vi "Init.vi"(8 "error in (no error)":errorcluster, 11 "Initial Data":string[][](table)=[["Test", "Dummy"], ["Operator", "John"], ["DUT", "Golden"], ["Serial Number", "0xAB"], ["Timestamp", "5/1/2023"]]) -> (0 "error out":errorcluster, 3 "DVR out":refnum<class "Data Server.lvclass">)   [LabVIEW 2021, in "Veristandgrpc_server.lvlib" / "Data Server.lvclass"]
uses:
  Data Server.lvclass
  Data Server.lvclass/Data Server.ctl
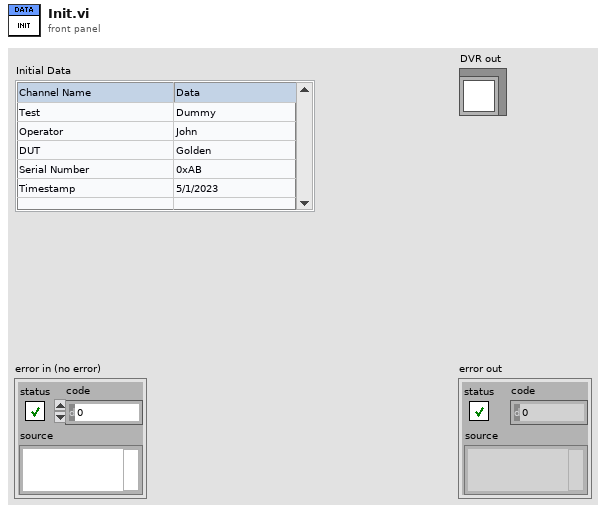
[diagram p1: front panel]
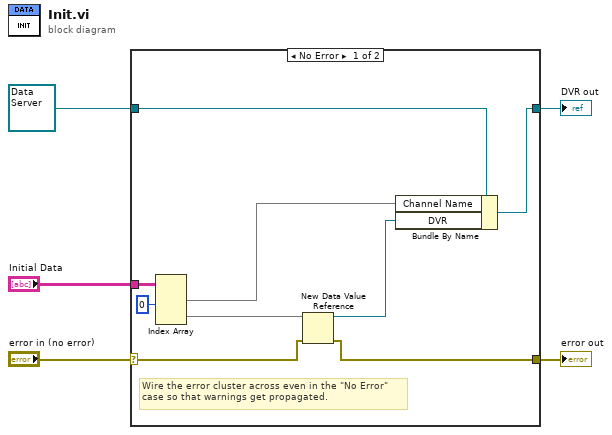
[diagram p0: block diagram]
diagram:
  n1 = case shown="No Error" "error in (no error)" {
    selector: "error in (no error)" -> [w9 w16]
    tunnel: [w7 w16] -> w4
    tunnel: [w13 w15] -> w2
    tunnel: refnum<class "Data Server.lvclass"> refnum ("DVR in") -> [w14 w15]
    tunnel: "Initial Data" -> [w12 _]
    frame No Error {
      # "Wire the error cluster across even in the \"No Error\"\ncase so that warnings get propagated."
      n2 = Index Array(array=w12, index (col) #1=0 ("disabled index (col)")) -> (element #1=w11:string[], element #2=w8:string[])  [unwired: 3 in]
      n3 = New Data Value Reference(data value=w8, error in=w9) -> (data value reference=w10:refnum<data-value>, error out=w7:errorcluster)
      n4 = Bundle By Name(cluster=w14, "Channel Name"=w11, "DVR"=w10) -> (w13:refnum<class "Data Server.lvclass">)
    }
    frame Error {
    }
  }
  "error out" <- w4
  "DVR out" <- w2
